vi "Write Overlay colors.vi"(8 "error in (no error)":errorcluster, 10 "Overlay colors":cluster{"Border":u32, "Text":u32}={"Border"=16448250, "Text"=16448250}, 11 "Overlay Base in":refnum<class "Analyze Results Base.lvclass">) -> (0 "error out":errorcluster, 3 "Overlay Base out":refnum<class "Analyze Results Base.lvclass">)   [LabVIEW 2014, in "Analyze Results Base.lvclass"]
uses:
  Analyze Results Base.lvclass
  Analyze Results Base.lvclass/Analyze Results Base.ctl
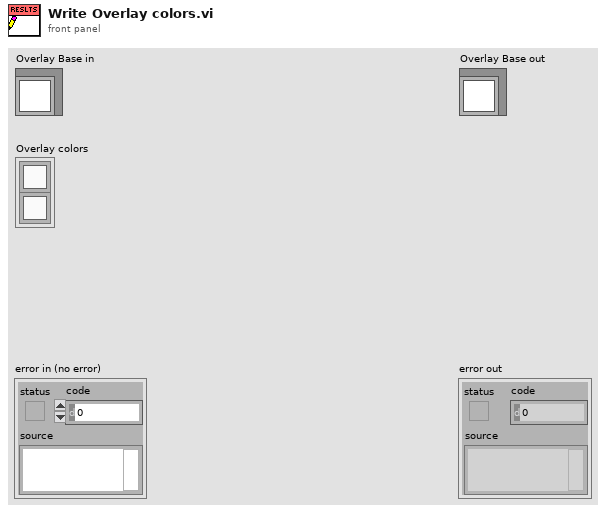
[diagram p1: front panel]
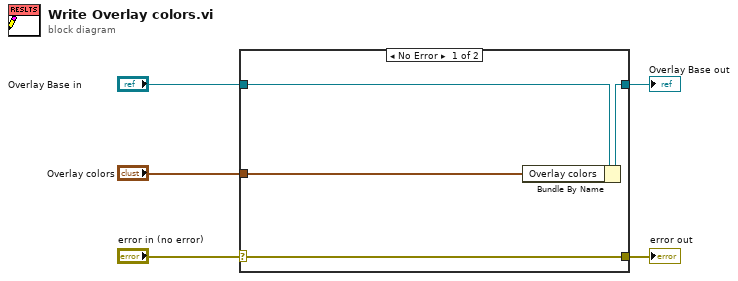
[diagram p0: block diagram]
diagram:
  n1 = case shown="No Error" "error in (no error)" {
    selector: "error in (no error)" -> [w9 w10]
    tunnel: [w9 w10] -> w4
    tunnel: [w7 w11] -> w2
    tunnel: "Overlay Base in" -> [w8 w11]
    tunnel: "Overlay colors" -> [w6 _]
    frame No Error {
      n2 = Bundle By Name(cluster=w8, "Overlay colors"=w6) -> (w7:refnum<class "Analyze Results Base.lvclass">)
    }
    frame Error {
    }
  }
  "error out" <- w4
  "Overlay Base out" <- w2
